vi "Setup AB Tovey.vi"(8 "error in (no error)":errorcluster, 10 "Model in":refnum<class "Model.lvclass">, 11 "Boot Loader in":refnum<class "Boot Loader.lvclass">) -> (0 "error out":errorcluster, 2 "Model out":refnum<class "Model.lvclass">, 3 "Boot Loader out":refnum<class "Boot Loader.lvclass">)   [LabVIEW 2015, in "Boot Loader.lvclass"]
uses:
  Boot Loader.lvclass
  Model/Model.lvclass
  <userlib>/Common/SerialProtocols/SerialProtocolFactory/SerialProtocolFactory/SerialProtocolFactory.lvclass
  <userlib>/Common/SerialProtocols/SerialCommunicator/SerialCommunicator.lvclass
  TEI-9150/Tovey 9150.lvclass
  <userlib>/Common/SerialProtocols/SerialCommunicator/SerialCommunicator.lvclass/SerialCommunicator.ctl
  TEI-9150/Tovey 9150.lvclass/Tovey 9150.ctl
  Model/Model.lvclass/Model.ctl
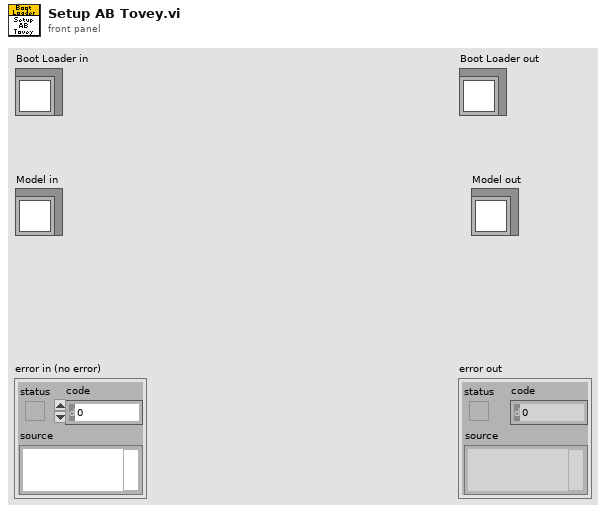
[diagram p1: front panel]
types:
  T1 = typedef "SerialProtocols.lvlib/SerialConfig.ctl" = cluster{"Serial Protocol":T2, "Protocol Parameters":T3, "Serial Message Parameters":T4}
  T2 = typedef "SerialProtocols.lvlib/SerialProtocol.ctl" = enum16{"RS232", "RS485", "SerialSimulator"}
  T3 = typedef "SerialProtocols.lvlib/ProtocolParameters.ctl" = cluster{"VISA resource name":refnum<visa-resource-name>, "Baud Rate":u32, "Data Bits":u16, "Parity":enum16{"None", "Odd", "Even", "Mark", "Space"}, "Flow Control":u16, "Stop Bits":u16, "Timeout (ms)":u32}
  T4 = typedef "SerialProtocols.lvlib/SerialMessageParameters.ctl" = cluster{"Byte Count":u32, "Enable Termination Character":bool, "Termination Char":u8}
  T5 = typedef "FAMT Typedefs.lvlib/Connection Settings.ctl" = cluster{"Pressure Servo Valve 1 DAC":u8, "Pressure Servo Valve 2 DAC":u8, "Flow Control Valve DAC":u8, "Load Cell ADC":u8, "FC1 ILC Port":refnum<visa-resource-name>, "FC2 ILC Port":refnum<visa-resource-name>, "Tovey A-B Port":refnum<visa-resource-name>, "Tovey C-D Port":refnum<visa-resource-name>, "Tovey E-F Port":refnum<visa-resource-name>, "FC1 ILC Protocol":T2, "FC2 ILC Protocol":T2, "Tovey A-B Protocol":T2, "Tovey C-D Protocol":T2, "Tovey E-F Protocol":T2, "Tovey A-B Address":u8, "Tovey C-D Address":u8, "Tovey E-F Address":u8}
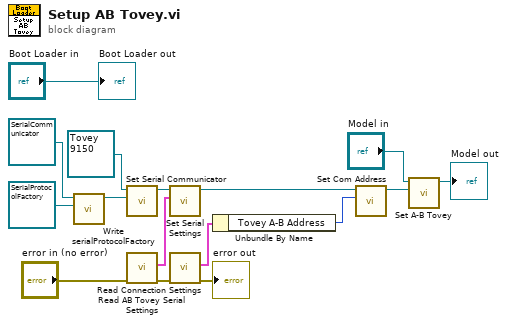
[diagram p0: block diagram]
diagram:
  n1 = call <userlib>:"Write serialProtocolFactory.vi"("serialProtocolFactory"=refnum<class "SerialProtocolFactory.lvclass"> refnum ("SerialCommFactory.lvclass"), "SerialCommunicator in"=refnum<class "SerialCommunicator.lvclass"> refnum ("SerialProtocols.lvlib:SerialCommunicator.lvclass")) -> ("SerialCommunicator out"=w13:refnum<class "SerialCommunicator.lvclass">)  [unwired: 9 in]
  n2 = call "Set Serial Communicator.vi"("SerialProtocols.lvlib:SerialCommunicator.lvclass"=w13, "Tovey9150 in"=refnum<class "Tovey 9150.lvclass"> refnum ("Tovey 9150.lvclass")) -> ("Tovey9150 out"=w11:refnum<class "Tovey 9150.lvclass">)  [unwired: 9 in]
  n3 = call "Read AB Tovey Serial Settings.vi"("error in (no error)"="error in (no error)") -> ("error out"=w7:errorcluster, "Serial"=w4:T1)  [unwired: 8 in, 1 out]
  n4 = call "Set Serial Settings.vi"("Serial Settings"=w4, "Tovey9150 in"=w11) -> ("Tovey9150 out"=w10:refnum<class "Tovey 9150.lvclass">)  [unwired: 9 in]
  n5 = call "Read Connection Settings.vi"("error in (no error)"=w7) -> ("error out"=→"error out":errorcluster, "Connection Settings"=w9:T5)  [unwired: 8 in, 1 out]
  n6 = Unbundle By Name(w9) -> ("Tovey A-B Address"=w8:u8)
  n7 = call "Set Com Address.vi"("Com Address"=w8, "Tovey9150 in"=w10) -> ("Tovey9150 out"=w1:refnum<class "Tovey 9150.lvclass">)  [unwired: 9 in]
  n8 = call "Set A-B Tovey.vi"("A-B Tovey"=w1, "Model in"="Model in") -> ("Model out"=→"Model out":refnum<class "Model.lvclass">)  [unwired: 9 in]
  "Boot Loader out" <- "Boot Loader in"
